vi "PreLoop.vi"(8 "error in":errorcluster, 11 "VI Ref":refnum<vi>) -> (0 "error out":errorcluster, 3 "Event Out":refnum<event-registration>)   [LabVIEW 2018, in "GUI3.lvclass"]
uses:
  GUI3.lvclass
  Queue/Queue.ctl
  Controller/GUI.lvclass
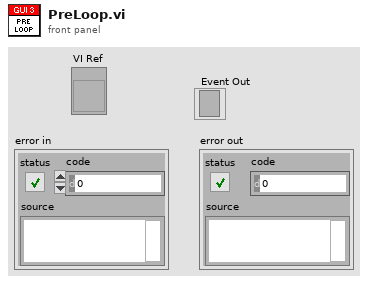
[diagram p1: front panel]
types:
  T1 = typedef "GUI3.lvclass/Queue.ctl" = enum16{"Create", "Get", "Destroy"}
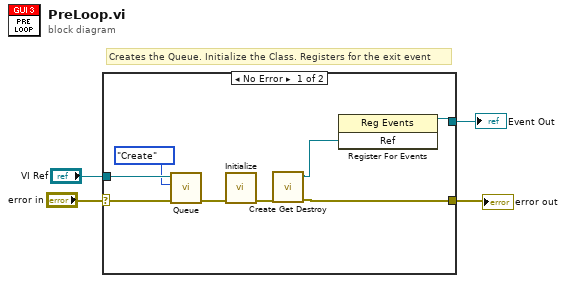
[diagram p0: block diagram]
diagram:
  # "Creates the Queue. Initialize the Class. Registers for the exit event"
  n1 = case shown="No Error" "error in" {
    selector: "error in" -> [w11 _]
    tunnel: [w6 _] -> w4
    tunnel: [w12 _] -> w1
    tunnel: "VI Ref" -> [w10 _]
    frame No Error {
      n2 = call "Queue.vi"("error in"=w11, "State(Get)"=Queue."Create" ("State"), "VI Ref"=w10) -> ("error out"=w8:errorcluster)  [unwired: 7 in, 1 out]
      n3 = call "Initialize.vi"("error in"=w8) -> ("error out"=w7:errorcluster)  [unwired: 10 in]
      n4 = call "Create Get Destroy.vi"("error In"=w7) -> ("Error Out"=w6:errorcluster, "Ref"=w5:refnum<user-event>)  [unwired: 9 in]
      n5 = register-events(w5) -> (reference out=w12:refnum<event-registration>)  [unwired: 2 in, 1 out]
    }
    frame Error {
    }
  }
  "error out" <- w4
  "Event Out" <- w1
